vi "Set freq pow and Ch.vi"(7 "Frequency Hz":dbl format="%#_13g", 8 "error in (no error)":errorcluster, 9 "On/Off":bool, 10 "Power lvl":dbl format="%#_13g", 11 "Channel":i32(ring)=1 items=["1"=1, "2"=2]) -> (0 "error out":errorcluster, 3 "resulting string":string)   [LabVIEW 2022 SP3, in "THz source modeule.lvlib"]
uses:
  THz source modeule.lvlib
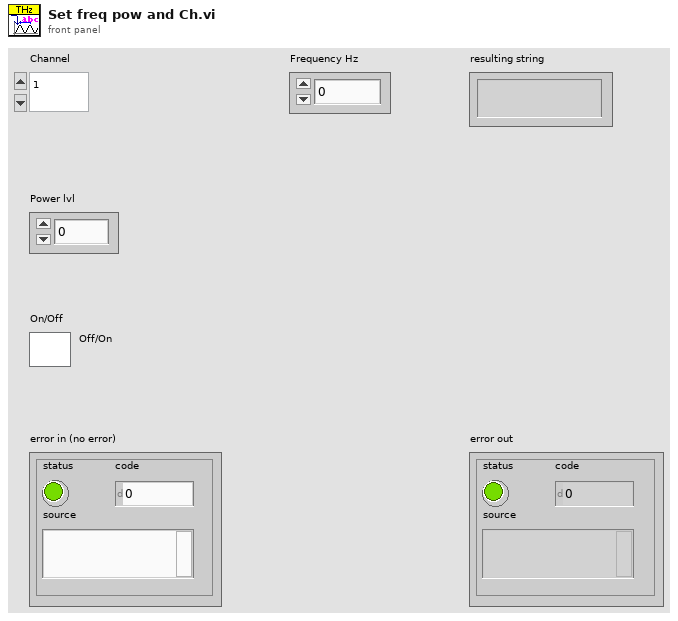
[diagram p1: front panel]
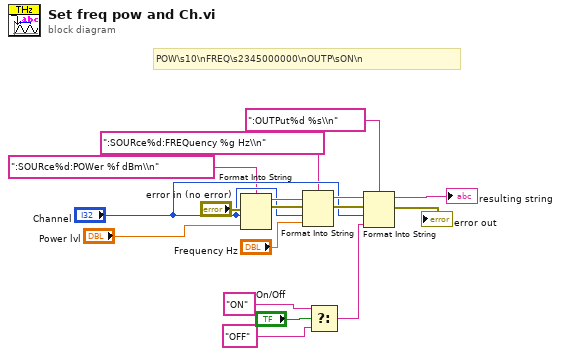
[diagram p0: block diagram]
diagram:
  # "POW\\s10\\nFREQ\\s2345000000\\nOUTP\\sON\\n"
  n1 = Format Into String(format string=":SOURce%d:POWer %f dBm\\n", error in="error in (no error)", "Channel", "Power lvl") -> (resulting string=w8:string, error out=w7:errorcluster)  [unwired: 1 in]
  n2 = Format Into String(format string=":SOURce%d:FREQuency %g Hz\\n", initial string=w8, error in=w7, "Channel", "Frequency Hz") -> (resulting string=w9:string, error out=w10:errorcluster)
  n3 = Select(t="ON", s="On/Off", f="OFF") -> (s? t:f=w14:string)
  n4 = Format Into String(format string=":OUTPut%d %s\\n", initial string=w9, error in=w10, "Channel", w14) -> (resulting string=→"resulting string":string, error out=→"error out":errorcluster)
